vi "Write SkillStateMachineRef.vi"(8 "error in (no error)":errorcluster, 10 "SkillStateMachine":refnum<class "SkillStateMachine.lvclass">, 11 "Tactic in":refnum<class "Tactic.lvclass">) -> (0 "error out":errorcluster, 3 "Tactic out":refnum<class "Tactic.lvclass">)   [LabVIEW 2018, in "Tactic.lvclass"]
uses:
  Tactic.lvclass
  SkillStateMachine_class/SkillStateMachine.lvclass
  Tactic.lvclass/Tactic.ctl
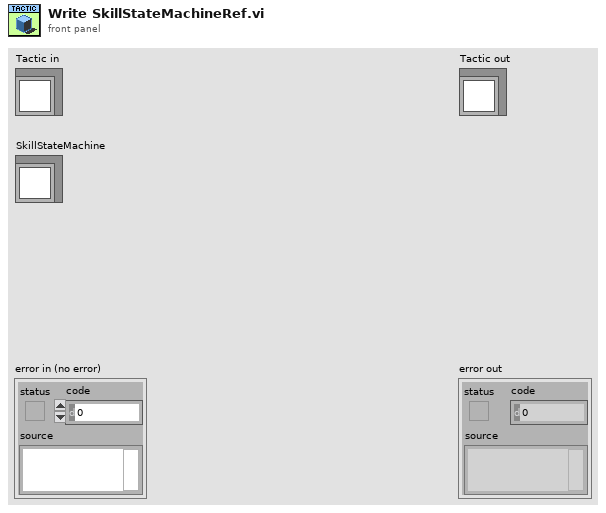
[diagram p1: front panel]
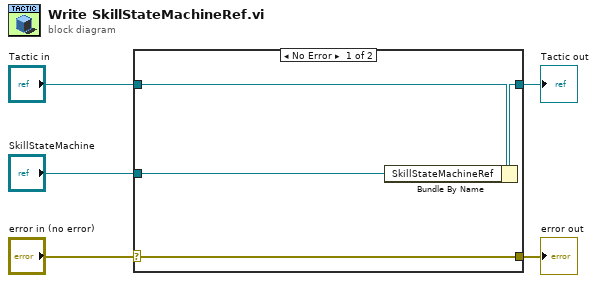
[diagram p0: block diagram]
diagram:
  n1 = case shown="No Error" "error in (no error)" {
    selector: "error in (no error)" -> [w9 w10]
    tunnel: [w9 w10] -> w4
    tunnel: [w7 w11] -> w2
    tunnel: "Tactic in" -> [w8 w11]
    tunnel: "SkillStateMachine" -> [w6 _]
    frame No Error {
      n2 = Bundle By Name(cluster=w8, "SkillStateMachineRef"=w6) -> (w7:refnum<class "Tactic.lvclass">)
    }
    frame Error {
    }
  }
  "error out" <- w4
  "Tactic out" <- w2
